vi "CH2_Comm_TCPIP.vi"() -> ()   [LabVIEW 2018]
uses:
  TCPIP/TCPIP.lvclass
  RxTx/RxTx.lvclass
panel:
  out "error out":errorcluster
  in  "RxTx.lvclass":refnum<class "RxTx.lvclass">
  in  "TCPIP.lvclass":refnum<class "TCPIP.lvclass">
  in  "Channel:":u16=2
  in  "Remote port":u16=59042
  # "Channel 2 - TCPIP Communication"
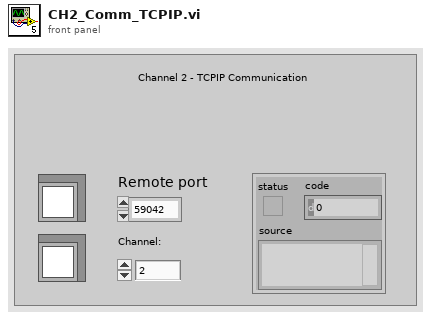
[diagram p1: front panel]
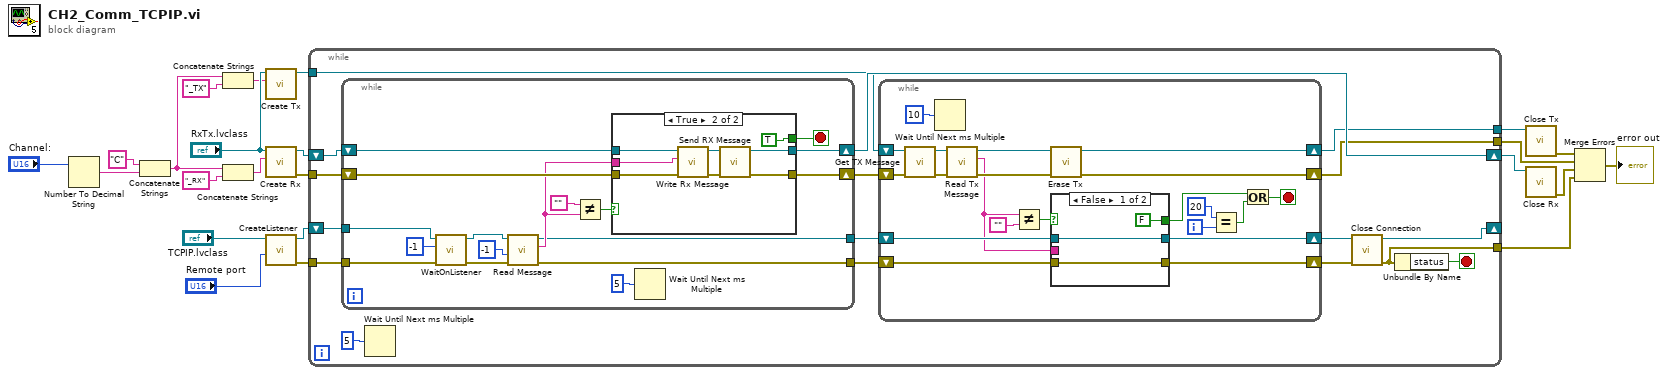
[diagram p0: block diagram]
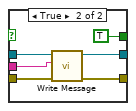
[diagram p2: hidden frame]
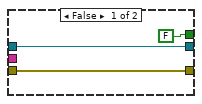
[diagram p3: hidden frame]
diagram:
  n1 = Number To Decimal String(number="Channel:") -> (decimal integer string=w19:string)  [unwired: 1 in]
  n2 = Concatenate Strings("C", w19) -> (w1:string)
  n3 = Concatenate Strings(w1, "_TX" ("Reader Name")) -> (w2:string)
  n4 = Concatenate Strings(w1, "_RX" ("Reader Name")) -> (w16:string)
  n5 = call "Create Tx.vi"("Writer Name"=w2, "RxTx in"="RxTx.lvclass") -> ("RxTx out"=w5:refnum<class "RxTx.lvclass">)  [unwired: 8 in, 1 out]
  n6 = call "Create Rx.vi"("Reader Name"=w16, "RxTx in"="RxTx.lvclass") -> ("error out"=w20:errorcluster, "RxTx out"=w14:refnum<class "RxTx.lvclass">)  [unwired: 8 in]
  n7 = call-dynamic "CreateListener.vi"("remote port"="Remote port", "TCPIP in"="TCPIP.lvclass") -> ("error out"=w21:errorcluster, "TCPIP out"=w11:refnum<class "TCPIP.lvclass">)  [unwired: 8 in]
  n8 = while {
    tunnel: w21 -> [w40]
    tunnel: w20 -> [w39]
    tunnel: w5 -> [w25]
    shift-right: [w36] -> w13
    shift-left: w14 -> [w37]
    tunnel: [w35] -> w12
    tunnel: [w34] -> w10
    tunnel: [w27] -> w7
    shift-right: [w29] -> _
    shift-left: w11 -> [w28]
    stop <- w26 stop-if-true
    n9 = while {
      shift-right: [w75] -> w24
      shift-left: w39 -> [w87]
      shift-right: [w76] -> w36
      shift-left: w37 -> [w86]
      tunnel: w28 -> [w80]
      tunnel: w40 -> [w79]
      tunnel: [w73] -> w33
      tunnel: [w72] -> w32
      stop <- w74 stop-if-true
      n10 = call-dynamic "WaitOnListener.vi"("error in (no error)"=w79, "timeout ms"=-1, "TCPIP in"=w80) -> ("error out"=w77:errorcluster, "TCPIP out"=w78:refnum<class "TCPIP.lvclass">)  [unwired: 7 in]
      n11 = call "Read Message.vi"("error in (no error)"=w77, "timeout"=-1, "TCPIP in"=w78) -> ("error out"=w72:errorcluster, "Message"=w82:string, "TCPIP out"=w73:refnum<class "TCPIP.lvclass">)  [unwired: 6 in]
      n12 = Not Equal?(x="", y=w82) -> (x != y?=w84:bool)
      n13 = case shown="True" w84 {
        tunnel: w87 -> [w89 w96]
        tunnel: w86 -> [w90 w95]
        tunnel: [w90 w93] -> w76
        tunnel: [w89 w92] -> w75
        tunnel: w82 -> [_ w94]
        tunnel: [FALSE TRUE] -> w74
        frame False {
        }
        frame True {
          n14 = call "Write Rx Message.vi"("error in (no error)"=w96, "Rx Message"=w94, "RxTx in"=w95) -> ("error out"=w97:errorcluster, "RxTx out"=w98:refnum<class "RxTx.lvclass">)  [unwired: 7 in]
          n15 = call "Send RX Message.vi"("error in (no error)"=w97, "RxTx in"=w98) -> ("error out"=w92:errorcluster, "RxTx out"=w93:refnum<class "RxTx.lvclass">)  [unwired: 8 in]
        }
      }
      n16 = Wait Until Next ms Multiple(millisecond multiple=u32 5) -> ()  [unwired: 1 out]
    }
    n17 = Wait Until Next ms Multiple(millisecond multiple=u32 5) -> ()  [unwired: 1 out]
    n18 = while {
      shift-right: [w50] -> w31
      shift-left: w33 -> [w59]
      shift-right: [w49] -> w30
      shift-left: w32 -> [w58]
      shift-right: [w61] -> w35
      shift-left: w25 -> [w48]
      shift-right: [w60] -> w34
      shift-left: w24 -> [w47]
      i -> [w45]
      stop <- w41 stop-if-true
      n19 = call "Get TX Message.vi"("error in (no error)"=w47, "RxTx in"=w48) -> ("error out"=w57:errorcluster, "RxTx out"=w53:refnum<class "RxTx.lvclass">)  [unwired: 8 in]
      n20 = Wait Until Next ms Multiple(millisecond multiple=u32 10) -> ()  [unwired: 1 out]
      n21 = call "Read Tx Message.vi"("error in (no error)"=w57, "RxTx in"=w53) -> ("error out"=w54:errorcluster, "Tx Message"=w52:string, "RxTx out"=w55:refnum<class "RxTx.lvclass">)  [unwired: 7 in]
      n22 = Not Equal?(x=w52, y="") -> (x != y?=w51:bool)
      n23 = call "Erase Tx.vi"("error in (no error)"=w54, "RxTx in"=w55) -> ("error out"=w60:errorcluster, "RxTx out"=w61:refnum<class "RxTx.lvclass">)  [unwired: 8 in]
      n24 = case shown="False" w51 {
        tunnel: w52 -> [_ w70]
        tunnel: w59 -> [w64 w69]
        tunnel: w58 -> [w63 w68]
        tunnel: [w64 w67] -> w50
        tunnel: [w63 w66] -> w49
        tunnel: [FALSE TRUE] -> w43
        frame False {
        }
        frame True {
          n25 = call "Write Message.vi"("error in (no error)"=w68, "Message"=w70, "TCPIP in"=w69) -> ("error out"=w66:errorcluster, "TCPIP out"=w67:refnum<class "TCPIP.lvclass">)  [unwired: 7 in]
        }
      }
      n26 = Equal?(x=20, y=w45) -> (x = y?=w42:bool)
      n27 = Or(x=w43, y=w42) -> (x .or. y?=w41:bool)
    }
    n28 = call "Close Connection.vi"("error in (no error)"=w30, "TCPIP in"=w31) -> ("error out"=w27:errorcluster, "TCPIP out"=w29:refnum<class "TCPIP.lvclass">)  [unwired: 8 in]
    n29 = Unbundle By Name(w27) -> ("status"=w26:bool)
  }
  n30 = call "Close Tx.vi"("RxTx in"=w12) -> ("error out"=w8:errorcluster)  [unwired: 9 in, 1 out]
  n31 = call "Close Rx.vi"("RxTx in"=w13) -> ("error out"=w6:errorcluster)  [unwired: 9 in, 1 out]
  n32 = Merge Errors(w8, w10, w6, w7) -> (→"error out":errorcluster)
